vi "ParseSetTracepoints.vi"(8 "error in (no error)":errorcluster, 11 "message body":variant) -> (0 "error out":errorcluster, 3 "tracepoints":T1[](array[typedef]))   [LabVIEW 2017, in "TraceLogger.lvlib"]
uses:
  <vilib>/addons/TraceLogger/TraceLogger.lvlib
  <vilib>/addons/TraceLogger/controls/TracepointConfig.ctl
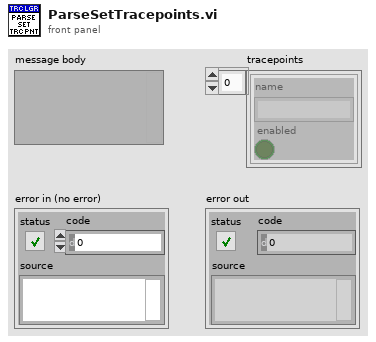
[diagram p1: front panel]
types:
  T1 = typedef "TraceLogger.lvlib/TracepointConfig.ctl" = cluster{"name":string, "enabled":bool}
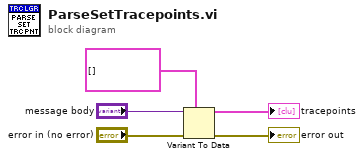
[diagram p0: block diagram]
diagram:
  n1 = Variant To Data(error in="error in (no error)", type=T1[] [] ("Tracepoints"), Variant="message body") -> (data=→"tracepoints":T1[], error out=→"error out":errorcluster)
